vi "Waterfall Global.vi"() -> ()   [LabVIEW 2024, in "Waterfall.lvlib" / "Waterfall.lvclass"]
uses:
  Waterfall.lvclass
panel:
  in  "Data to Process":string="Data to process (s)"
  in  "Show Waterfall Plot":string="Show waterfall plot"
  in  "Number of averages":string="Number of averages"
  in  "Weighting Mode":string="Weighting mode"
  in  "Weighting Mode Options":string[](array[string])=["Linear", "Exponential"]
  in  "Averaging Mode":string="Averaging mode"
  in  "Averaging Mode Options":string[](array[string])=["No averaging", "Vector averaging", "RMS averaging", "Peak hold"]
  in  "Window":string="Window"
  in  "Window Options":string[](array[string])=["Rectangle", "Hanning", "Hamming", "Blackman-Harris", "Exact Blackman", "Blackman", "Flat Top", "4 Term B-Harris", "7 Term B-Harris", "Low Sidelobe", "Blackman Nuttal", "Triangle", "Barlett-Hanning", "Bohman", "Parzen", "Welch", "Kaiser", "Dolph-Chebychev", "Gaussian"]
  in  "Slice":string="Slice (s)"
  in  "Select channel":string="Select channel"
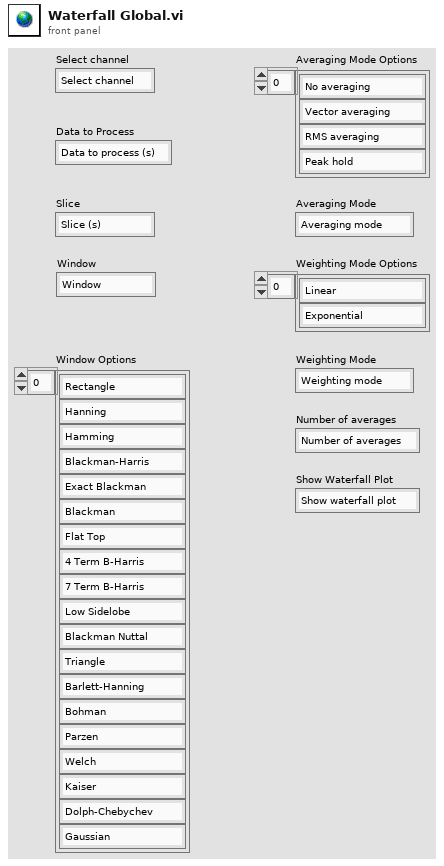
[diagram p1: front panel]
diagram:
